vi "EditorPDF closePDF.vi"(8 "error in (no error)":errorcluster, 11 "CreatePDF in":refnum<class "CreatePDF.lvclass">) -> (0 "error out":errorcluster, 3 "CreatePDF out":refnum<class "CreatePDF.lvclass">)   [LabVIEW 2018, in "CreatePDF.lvclass"]
uses:
  CreatePDF.lvclass
  CreatePDF.lvclass/CreatePDF.ctl
  <vilib>/Simplicity AI/SAI_PDF_API/Classes/Context/Context.lvclass
  <vilib>/Simplicity AI/SAI_PDF_API/SAI_PDF_Toolkit.lvlib
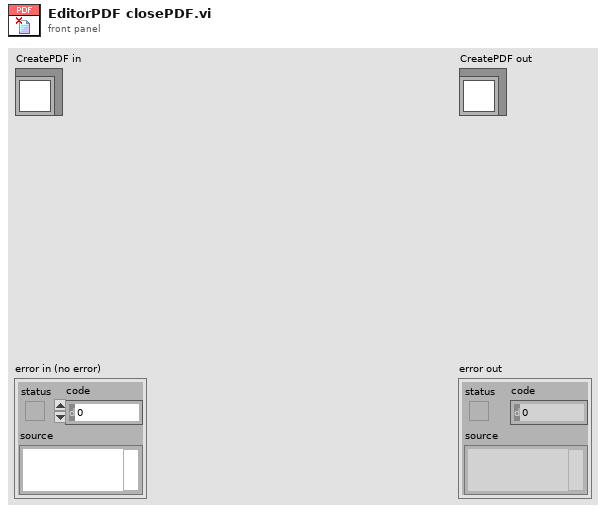
[diagram p1: front panel]
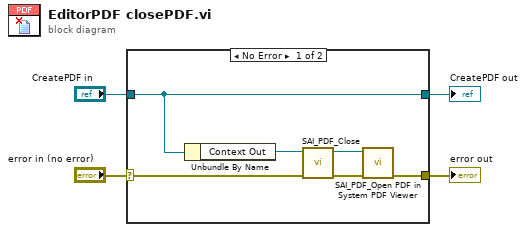
[diagram p0: block diagram]
diagram:
  n1 = case shown="No Error" "error in (no error)" {
    selector: "error in (no error)" -> [w5 w12]
    tunnel: [w6 w12] -> w3
    tunnel: [w8 w11] -> w1
    tunnel: "CreatePDF in" -> [w8 w11]
    frame No Error {
      n2 = Unbundle By Name(w8) -> ("Context Out"=w7:refnum<class "Context.lvclass">)
      n3 = call <vilib>:"SAI_PDF_Close.vi"("error in"=w5, "Context In"=w7) -> ("error out"=w9:errorcluster, "Path"=w10:path)  [unwired: 8 out]
      n4 = call <vilib>:"SAI_PDF_Open PDF in System PDF Viewer.vi"("error in"=w9, "Path"=w10) -> ("error out"=w6:errorcluster)  [unwired: 9 out]
    }
    frame Error {
    }
  }
  "error out" <- w3
  "CreatePDF out" <- w1
